vi "Tx Buffered Packet Page.vi"(8 "error in (no error)":errorcluster, 11 "Node Ptr":T6 format="%.0x") -> (0 "error out":errorcluster)   [LabVIEW 2019, in "UDP-Custom-Device System Explorer.lvlib"]
uses:
  UDP-Custom-Device System Explorer.lvlib
  Shared/Types/Shared - Transmit Sim Options.ctl
  Shared/Types/Shared - Transmit Flag Options.ctl
  Shared/Types/Shared - Transmit Echo Options.ctl
  Shared/Types/Shared - Transmit Buffer Options.ctl
  Shared/Types/Shared - Pointer Encoding.ctl
  <vilib>/NI VeriStand/Custom Device API/Custom Device Item Ref.ctl
  Types/Page References/Refs - Tx Buffered Data Packet Page.ctl
  <vilib>/NI VeriStand/Custom Device API/Custom Device API.lvlib
  Property Accessors/Shared Packet Accessors.lvlib
  Property Accessors/Tx Packet Accessors.lvlib
  Property Accessors/Buffered Data Packet.lvlib
  Shared/UDP-Custom-Device Shared.lvlib
panel:
  in  "Config Threading":bool
  in  "Toggle Sim":bool
  in  "Sim Options":T1
  in  "Buffer Options":T2
  in  "Debug Mode":bool caption="Auto-Assign Local NIC"
  in  "Transmit Echo Options":T3
  in  "Transmit Options":T4=enum."One-Shot"
  in  "Port as Channel?":bool caption="Auto-Assign Local NIC"
  in  "Pointer Encoding":T5
  in  "TTL":u16=1
  in  "Multicast?":bool caption="Auto-Assign Local NIC"
  in  "External Buffer?":bool
  in  "Buffer Size (bytes)":u32
  in  "General Header 3":cluster{"Section Name":string}={"Section Name"="Buffer Configuration"}
  in  "Prepend\nHeader?":bool caption="Auto-Assign Local NIC"
  in  "Auto-Assign Local NIC":bool
  in  "Port":u16
  in  "IP Address of Local NIC":string
  in  "General Header 2":cluster{"Section Name":string}={"Section Name"="Network Settings"}
  in  "Destination Port":u16
  in  "IP Address of Destination":string
  in  "Configure Header":bool
  in  "Endianness":u16(ring) items=["big-endian"=0, "little-endian"=2]
  out "Packet ID":i32
  in  "Description":string
  in  "Name":string
  in  "SHDocVw.IWebBrowser":refnum<k7>(container)
  in  "General Header":cluster{"Section Name":string}={"Section Name"="Buffered Transmit Packet"}
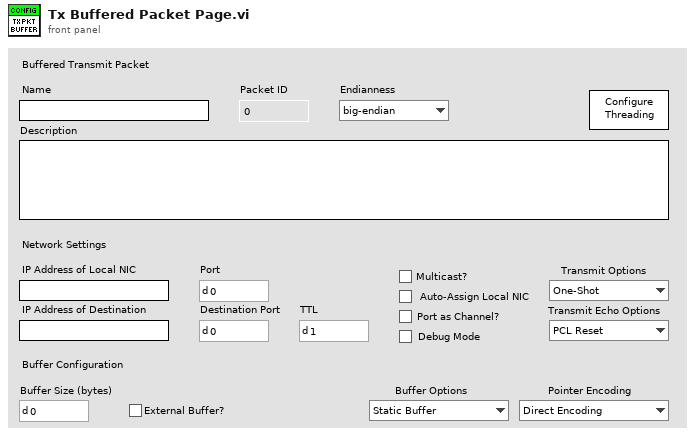
[diagram p1: front panel]
types:
  T1 = typedef "UDP-Custom-Device Shared.lvlib/Shared - Transmit Sim Options.ctl" = enum16{"No Simulation", "Counter", "Full Buffer", "FIFO Test", "FIFO + Port Test"}
  T2 = typedef "UDP-Custom-Device Shared.lvlib/Shared - Transmit Buffer Options.ctl" = enum16{"Static Buffer", "FIFO Buffer", "FIFO Buffer + Port"}
  T3 = typedef "UDP-Custom-Device Shared.lvlib/Shared - Transmit Echo Options.ctl" = enum16{"PCL Reset", "Counter", "Mirror"}
  T4 = typedef "UDP-Custom-Device Shared.lvlib/Shared - Transmit Flag Options.ctl" = enum16{"Always", "One-Shot", "Toggle"}
  T5 = typedef "UDP-Custom-Device Shared.lvlib/Shared - Pointer Encoding.ctl" = enum16{"Direct Encoding", "Conversion Encoding"}
  T6 = typedef "Custom Device API.lvlib/Custom Device Item Ref.ctl" = u64
  T7 = typedef "UDP-Custom-Device System Explorer.lvlib/Refs - Tx Buffered Data Packet Page.ctl" = cluster{"Name":refnum<vi>, "Description":refnum<vi>, "Packet ID":refnum<vi>, "Endianness":refnum<vi>, "Prepend\nHeader?":refnum<vi>, "Configure Header":refnum<vi>, "IP Address of Local NIC":refnum<vi>, "Port":refnum<vi>, "IP Address of Destination":refnum<vi>, "Destination Port":refnum<vi>, "Auto-Assign Local NIC":refnum<vi>, "External Buffer?":refnum<vi>, "Buffer Size (bytes)":refnum<vi>, "Multicast?":refnum<vi>, "TTL":refnum<vi>, "Pointer Encoding":refnum<vi>, "Port as Channel?":refnum<vi>, "Transmit Options":refnum<vi>, "Transmit Echo Options":refnum<vi>, "Debug Mode":refnum<vi>, "Buffer Options":refnum<vi>, "Sim Options":refnum<vi>}
  T8 = enum8{"Enabled", "Disabled", "Disabled and Grayed Out"}
  T9 = typedef "Custom Device API.lvlib/Custom Device Commands.ctl" = enum16{"Default", "Item renamed", "Shutdown", "Dynamic button pressed"}
  T10 = typedef "UDP-Custom-Device System Explorer.lvlib/Thread Configuration.ctl" = cluster{"targetProcessor":i8, "targetPriority":i16, "Synchronization":T11, "loopPeriod":u32, "pclDecimation":u16, "threadManagement":T12}
  T11 = typedef "UDP-Custom-Device System Explorer.lvlib/Thread Sync Reference.ctl" = enum16{"PCL", "Async"}
  T12 = typedef "UDP-Custom-Device Shared.lvlib/Shared - Thread Management.ctl" = enum16{"Untimed (Default)", "Timed (High Priority)"}
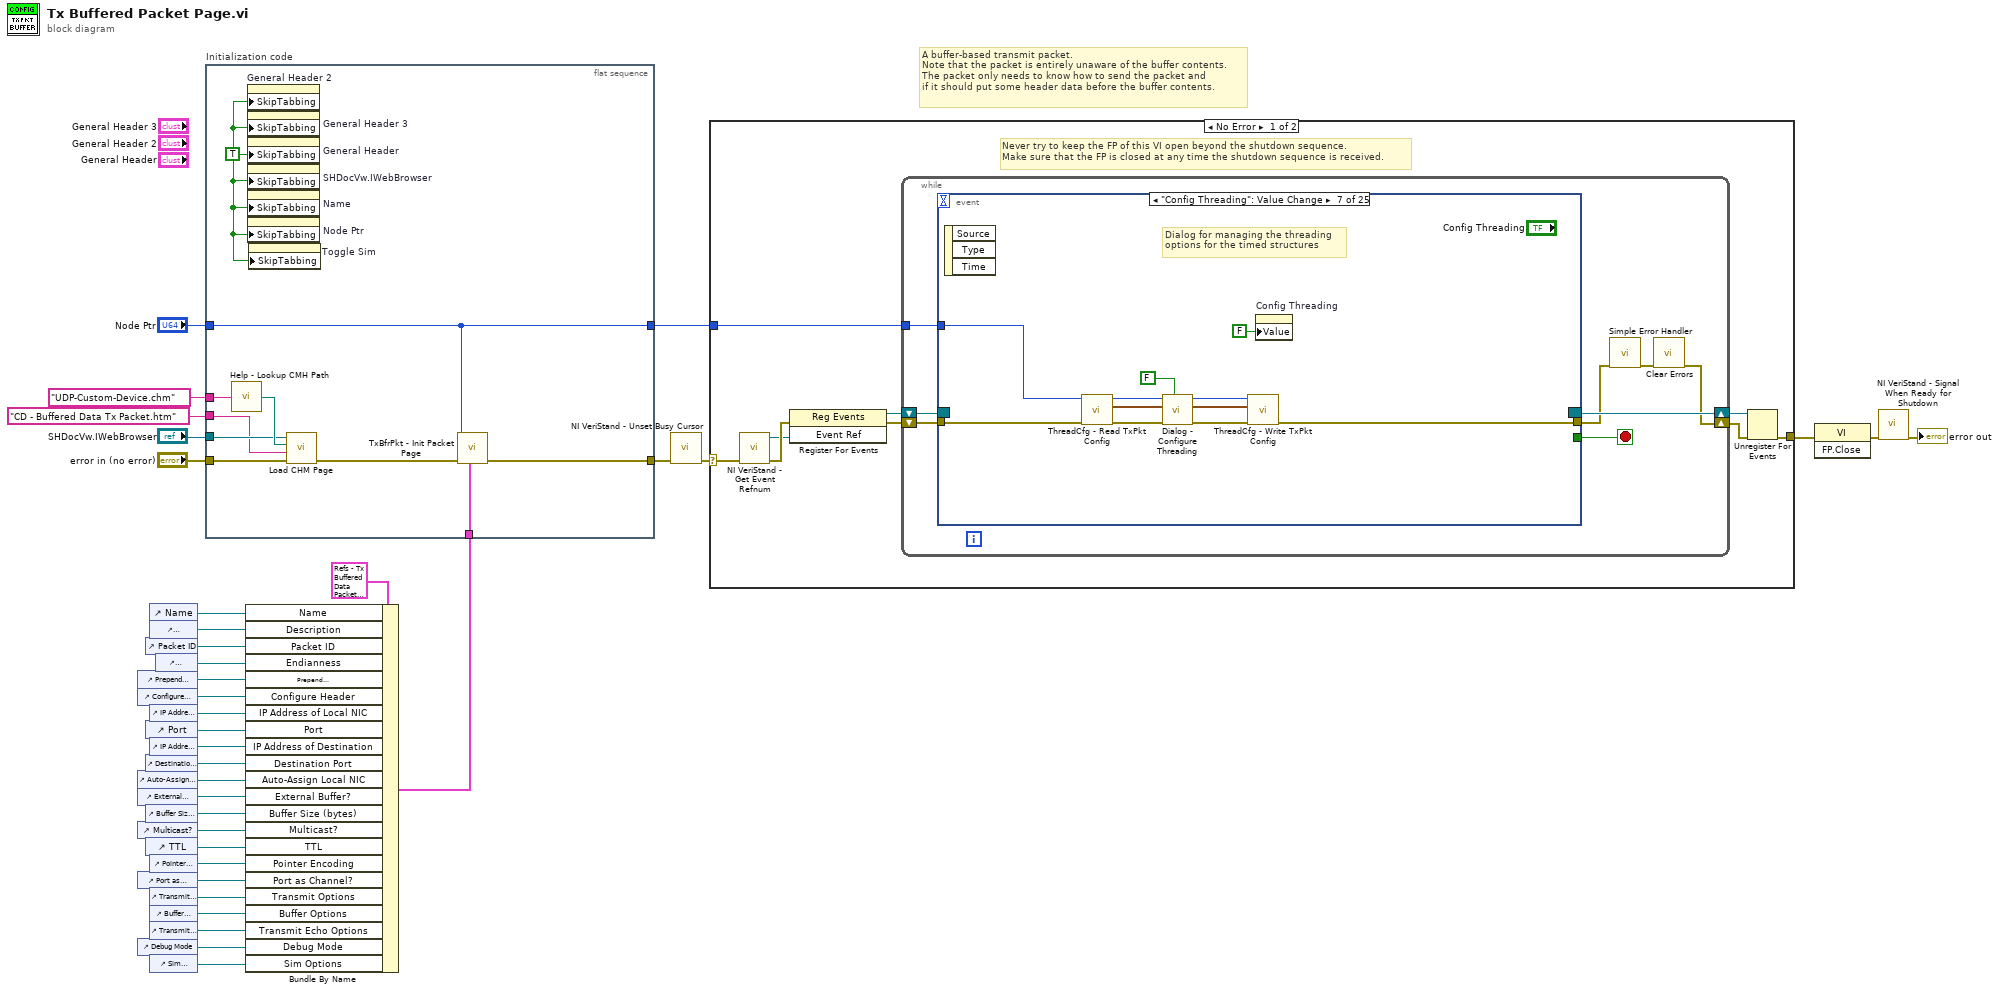
[diagram p0: block diagram]
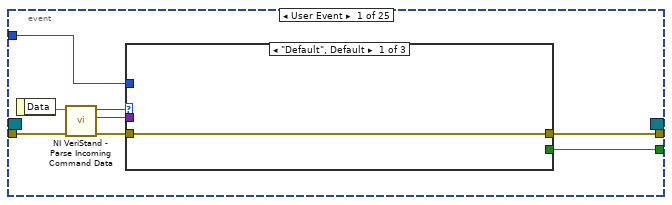
[diagram p2: hidden frame]
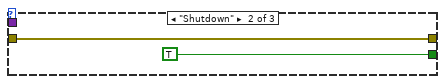
[diagram p3: hidden frame]
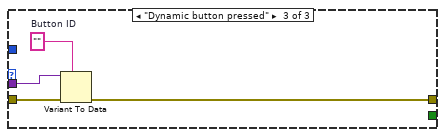
[diagram p4: hidden frame]
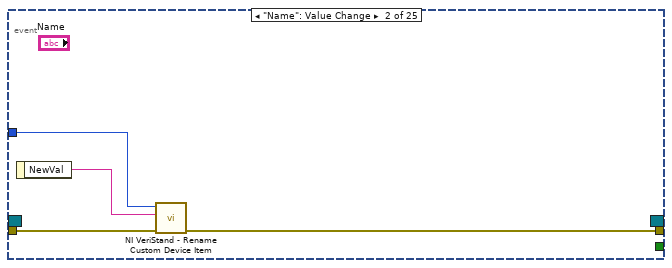
[diagram p5: hidden frame]
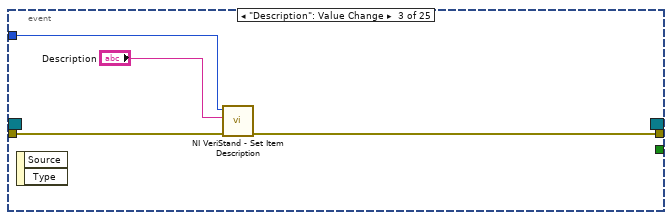
[diagram p6: hidden frame]
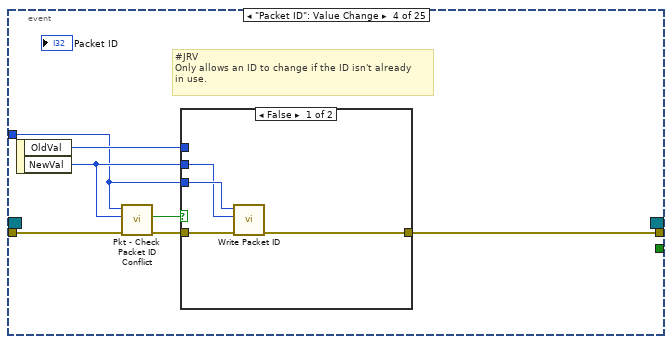
[diagram p7: hidden frame]
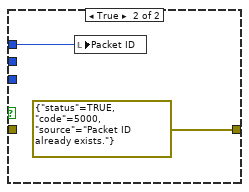
[diagram p8: hidden frame]
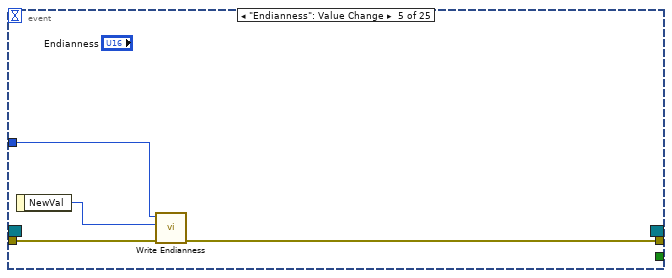
[diagram p9: hidden frame]
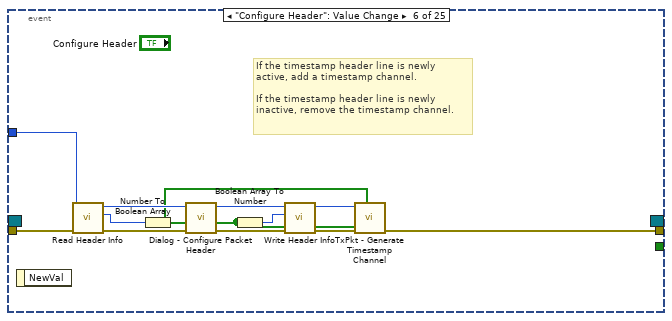
[diagram p10: hidden frame]
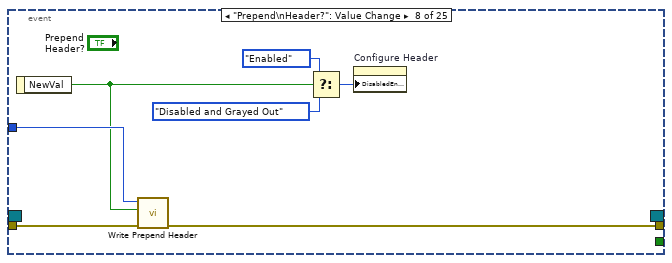
[diagram p11: hidden frame]
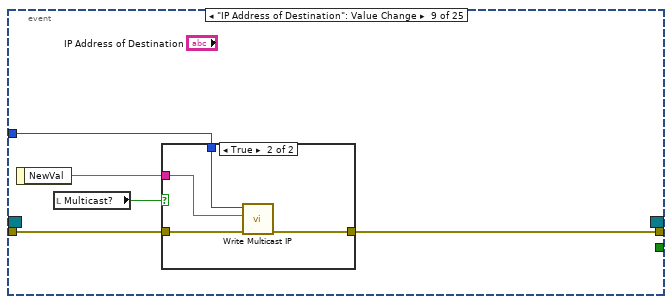
[diagram p12: hidden frame]
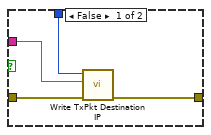
[diagram p13: hidden frame]
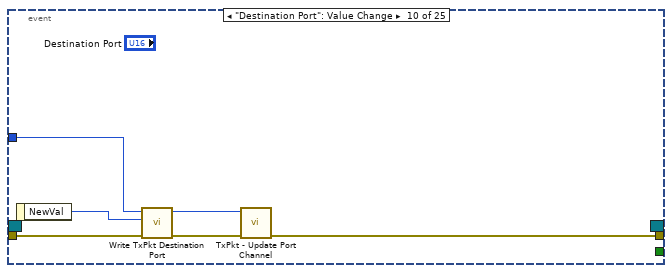
[diagram p14: hidden frame]
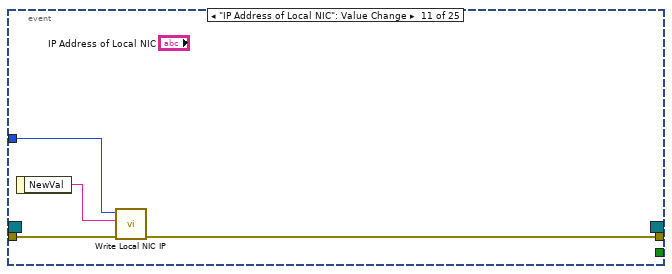
[diagram p15: hidden frame]
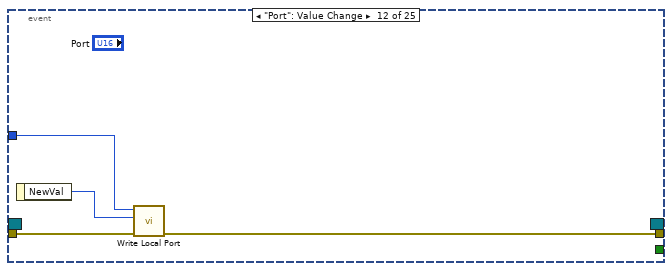
[diagram p16: hidden frame]
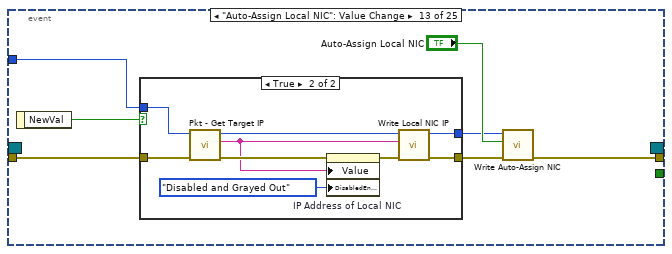
[diagram p17: hidden frame]
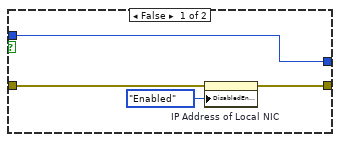
[diagram p18: hidden frame]
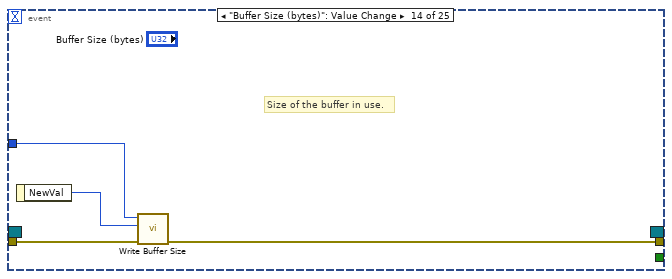
[diagram p19: hidden frame]
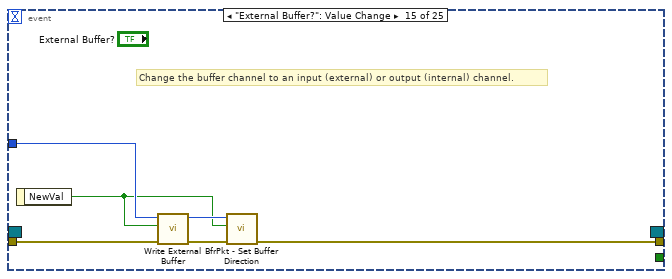
[diagram p20: hidden frame]
diagram:
  # "A buffer-based transmit packet.\nNote that the packet is entirely unaware of the buffer contents.\nThe packet only needs to know how to send the packet and\nif it should put some header data before the buffer contents."
  n1 = control-ref of="Prepend\nHeader?"() -> (w19:refnum<vi>)
  n2 = control-ref of="Configure Header"() -> (w18:refnum<vi>)
  n3 = control-ref of="Auto-Assign Local NIC"() -> (w13:refnum<vi>)
  n4 = control-ref of="External Buffer?"() -> (w12:refnum<vi>)
  n5 = control-ref of="Multicast?"() -> (w9:refnum<vi>)
  n6 = control-ref of="Port as Channel?"() -> (w6:refnum<vi>)
  n7 = control-ref of="Debug Mode"() -> (w3:refnum<vi>)
  n8 = control-ref of="Packet ID"() -> (w21:refnum<vi>)
  n9 = control-ref of="Port"() -> (w16:refnum<vi>)
  n10 = control-ref of="Destination Port"() -> (w14:refnum<vi>)
  n11 = control-ref of="Buffer Size (bytes)"() -> (w11:refnum<vi>)
  n12 = control-ref of="TTL"() -> (w8:refnum<vi>)
  n13 = control-ref of="Name"() -> (w23:refnum<vi>)
  n14 = control-ref of="Description"() -> (w22:refnum<vi>)
  n15 = control-ref of="IP Address of Local NIC"() -> (w17:refnum<vi>)
  n16 = control-ref of="IP Address of Destination"() -> (w15:refnum<vi>)
  n17 = control-ref of="Pointer Encoding"() -> (w7:refnum<vi>)
  n18 = control-ref of="Transmit Options"() -> (w5:refnum<vi>)
  n19 = control-ref of="Buffer Options"() -> (w2:refnum<vi>)
  n20 = control-ref of="Transmit Echo Options"() -> (w4:refnum<vi>)
  n21 = control-ref of="Sim Options"() -> (w1:refnum<vi>)
  n22 = control-ref of="Endianness"() -> (w20:refnum<vi>)
  n23 = flat-sequence "Initialization code" {
    tunnel: "error in (no error)" -> [w44]
    tunnel: "Node Ptr" -> [w40]
    tunnel: [w38] -> w31
    tunnel: [w40] -> w28
    tunnel: "SHDocVw.IWebBrowser" -> [w43]
    tunnel: "CD - Buffered Data Tx Packet.htm" ("CD_CHM_Section") -> [w41]
    tunnel: "UDP-Custom-Device.chm" ("CD_CHM_FileName") -> [w42]
    tunnel: w10 -> [w37]
    frame #0 {
      w36 = TRUE ("Skip When Tabbing")
      n24 = call "Help - Lookup CMH Path.vi"("Main CMH File"=w42) -> ("Compiled CMH Path"=w45:path)
      n25 = property on="General Header 2" class="Clust (strict)"("SkipTabbing"=w36) -> ()  [unwired: 2 in, 2 out]
      n26 = property on="General Header 3" class="Clust (strict)"("SkipTabbing"=w36) -> ()  [unwired: 2 in, 2 out]
      n27 = property on="General Header" class="Clust (strict)"("SkipTabbing"=w36) -> ()  [unwired: 2 in, 2 out]
      n28 = property on="SHDocVw.IWebBrowser" class="AXCont"("SkipTabbing"=w36) -> ()  [unwired: 2 in, 2 out]
      n29 = property on="Name" class="Str"("SkipTabbing"=w36) -> ()  [unwired: 2 in, 2 out]
      n30 = property on="Node Ptr" class="DigNum (strict)"("SkipTabbing"=w36) -> ()  [unwired: 2 in, 2 out]
      n31 = property on="Toggle Sim" class="Bool"("SkipTabbing"=w36) -> ()  [unwired: 2 in, 2 out]
      n32 = call <vilib>:"Load CHM Page.vi"("error in (no error)"=w44, "HTML File"=w41, "Compiled CHM Path"=w45, "Web Browser Reference"=w43) -> ("error out"=w39:errorcluster)  [unwired: 7 in]
      n33 = call "TxBfrPkt - Init Packet Page.vi"("Tx Buffered Data Packet Refs"=w37, "error in (no error)"=w39, "Node Ptr In"=w40) -> ("error out"=w38:errorcluster)  [unwired: 7 in, 1 out]
    }
  }
  n34 = Bundle By Name(cluster=T7 {"Name"=refnum, "Description"=refnum, "Packet ID"=refnum, "Endianness"=refnum, "Prepend\nHeader?"=refnum, "Configure Header"=refnum, "IP Address of Local NIC"=refnum, "Port"=refnum, "IP Address of Destination"=refnum, "Destination Port"=refnum, "Auto-Assign Local NIC"=refnum, "External Buffer?"=refnum, "Buffer Size (bytes)"=refnum, "Multicast?"=refnum, "TTL"=refnum, "Pointer Encoding"=refnum, "Port as Channel?"=refnum, "Transmit Options"=refnum, "Transmit Echo Options"=refnum, "Debug Mode"=refnum, "Buffer Options"=refnum, "Sim Options"=refnum} ("Tx Buffered Data Packet Refs"), "Name"=w23, "Description"=w22, "Packet ID"=w21, "Endianness"=w20, "Prepend\nHeader?"=w19, "Configure Header"=w18, "IP Address of Local NIC"=w17, "Port"=w16, "IP Address of Destination"=w15, "Destination Port"=w14, "Auto-Assign Local NIC"=w13, "External Buffer?"=w12, "Buffer Size (bytes)"=w11, "Multicast?"=w9, "TTL"=w8, "Pointer Encoding"=w7, "Port as Channel?"=w6, "Transmit Options"=w5, "Buffer Options"=w2, "Transmit Echo Options"=w4, "Debug Mode"=w3, "Sim Options"=w1) -> (w10:T7)
  n35 = call <vilib>:"NI VeriStand - Unset Busy Cursor.vi"("error in (no error)"=w31) -> ("error out"=w30:errorcluster)  [unwired: 10 out]
  n36 = case shown="No Error" w30 {
    selector: w30 -> [w46 w254]
    tunnel: [w51 w252] -> w35
    tunnel: w28 -> [w47 _]
    frame No Error {
      # "Never try to keep the FP of this VI open beyond the shutdown sequence.\nMake sure that the FP is closed at any time the shutdown sequence is received."
      n37 = call <vilib>:"NI VeriStand - Get Event Refnum.vi"("error in (no error)"=w46) -> ("error out"=w54:errorcluster, "Event Ref"=w50:refnum<user-event>)  [unwired: 9 out]
      n38 = register-events(error in=w54, w50) -> (reference out=w48:refnum<event-registration>, error out=w49:errorcluster)  [unwired: 1 in]
      n39 = while {
        tunnel: w47 -> [w58]
        shift-right: [w55] -> w52
        shift-left: w49 -> [w61]
        shift-right: [w62] -> w53
        shift-left: w48 -> [w60]
        stop <- w59 stop-if-true
        n40 = event shown="[6] \"Config Threading\": Value Change" {
          selector: w60 -> [_ _ _ _ _ _ _ _ _ _ _ _ _ _ _ _ _ _ _ _ _ _ _ _ _]
          dyn-events: [_ _ _ _ _ _ _ _ _ _ _ _ _ _ _ _ _ _ _ _ _ _ _ _ _] -> w62
          timeout: _ -> [_ _ _ _ _ _ _ _ _ _ _ _ _ _ _ _ _ _ _ _ _ _ _ _ _]
          tunnel: w61 -> [w70 w81 w85 w90 w102 w105 w126 w130 w136 w152 w154 w160 w167 w182 w189 w192 w200 w214 w221 w224 w228 w233 w242 w246 w249]
          tunnel: [w66 _ _ _ _ _ _ _ _ _ _ _ _ _ _ _ _ _ _ _ _ _ _ _ _] -> w59
          tunnel: [w65 w79 w82 w86 w99 w103 w117 w127 w135 w147 w153 w157 w162 w181 w186 w191 w195 w212 w216 w222 w226 w232 w241 w245 w249] -> w57
          tunnel: w58 -> [w64 w80 w84 w87 w101 w104 w125 w129 w138 w150 w155 w158 w165 w184 w190 w193 w201 w215 w219 w225 w229 w234 w244 w248 _]
          event User Event {
            n41 = event-data() -> ("Data"=w69:string)  [unwired: 1 out]
            n42 = call <vilib>:"NI VeriStand - Parse Incoming Command Data.vi"("error in (no error)"=w70, "Incoming data"=w69) -> ("error out"=w68:errorcluster, "Outgoing data"=w63:variant, "Action"=w67:T9)  [unwired: 7 out]
            n43 = case shown="\"Default\", Default" w67 {
              tunnel: w68 -> [w71 w72 w77]
              tunnel: [_ TRUE _] -> w66
              tunnel: [w71 w72 w74] -> w65
              tunnel: w64 -> [_ _ _]
              tunnel: w63 -> [_ _ w76]
              frame "Default", Default {
              }
              frame "Shutdown" {
              }
              frame "Dynamic button pressed" {
                w75 = ""  # Button ID
                n44 = Variant To Data(error in=w77, type=w75, Variant=w76) -> (error out=w74:errorcluster)  [unwired: 1 out]
              }
            }
          }
          event "Name": Value Change {
            n45 = event-data() -> ("NewVal"=w78:string)  [unwired: 1 out]
            n46 = call <vilib>:"NI VeriStand - Rename Custom Device Item.vi"("error in (no error)"=w81, "New Name"=w78, "Item Ref in"=w80) -> ("error out"=w79:errorcluster)  [unwired: 6 in, 2 out]
          }
          event "Description": Value Change {
            n47 = event-data() -> ()  [unwired: 3 out]
            n48 = call <vilib>:"NI VeriStand - Set Item Description.vi"("error in (no error)"=w85, "Description"="Description", "Item Ref in"=w84) -> ("error out"=w82:errorcluster)  [unwired: 6 in, 2 out]
          }
          event "Packet ID": Value Change {
            # "#JRV\nOnly allows an ID to change if the ID isn't already\nin use."
            n49 = event-data() -> ("OldVal"=w89:i32, "NewVal"=w88:i32)  [unwired: 1 out]
            n50 = call "Pkt - Check Packet ID Conflict.vi"("error in (no error)"=w90, "New ID"=w88, "Packet Ref In"=w87) -> ("error out"=w92:errorcluster, "Conflicting ID?"=w91:bool)  [unwired: 7 in]
            n51 = case shown="False" w91 {
              tunnel: w92 -> [w94 _]
              tunnel: w87 -> [w96 _]
              tunnel: [w93 errorcluster {"status"=TRUE, "code"=5000, "source"="Packet ID already exists."} ("error out")] -> w86
              tunnel: w89 -> [_ w97]
              tunnel: w88 -> [w95 _]
              frame False {
                n52 = call "Write Packet ID.vi"("error in (no error)"=w94, "Packet ID"=w95, "Node Ptr"=w96) -> ("error out"=w93:errorcluster)  [unwired: 7 in, 1 out]
              }
              frame True {
                n53 = local write "Packet ID"(w97) -> ()
              }
            }
          }
          event "Endianness": Value Change {
            n54 = event-data() -> ("NewVal"=w100:u16)  [unwired: 1 out]
            n55 = call "Write Endianness.vi"("error in (no error)"=w102, "Endianness"=w100, "Node Ptr"=w101) -> ("error out"=w99:errorcluster)  [unwired: 7 in, 1 out]
          }
          event "Configure Header": Value Change {
            # "If the timestamp header line is newly\nactive, add a timestamp channel.\n\nIf the timestamp header line is newly\ninactive, remove the timestamp channel."
            n56 = event-data() -> ()  [unwired: 2 out]
            n57 = call "Read Header Info.vi"("error in (no error)"=w105, "Node Ptr"=w104) -> ("error out"=w113:errorcluster, "Header Info"=w114:u32, "Node Ptr out"=w115:T6)  [unwired: 7 in]
            n58 = Number To Boolean Array(number=w114) -> (Boolean array=w106:bool[])
            n59 = call "Dialog - Configure Packet Header.vi"("error in (no error)"=w113, "Header Elements In"=w106, "Packet Ref in"=w115) -> ("error out"=w109:errorcluster, "Header Elements Out"=w107:bool[], "Packet Ref out"=w108:T6)  [unwired: 6 in]
            n60 = Boolean Array To Number(Boolean array=w107) -> (number=w110:u32)
            n61 = call "Write Header Info.vi"("error in (no error)"=w109, "Header Info"=w110, "Node Ptr"=w108) -> ("error out"=w112:errorcluster, "Node Ptr out"=w111:T6)  [unwired: 7 in]
            n62 = call "TxPkt - Generate Timestamp Channel.vi"("New Header Config"=w107, "Previous Header Config"=w106, "error in (no error)"=w112, "Packet Ref in"=w111) -> ("error out"=w103:errorcluster)  [unwired: 6 in, 1 out]
          }
          event "Config Threading": Value Change {
            # "Dialog for managing the threading\noptions for the timed structures"
            n63 = event-data() -> ()  [unwired: 4 out]
            n64 = call "ThreadCfg - Read TxPkt Config.vi"("error in (no error)"=w126, "Node Ptr In"=w125) -> ("error out"=w123:errorcluster, "threadOptions"=w121:T10, "Node Ptr Out"=w124:T6)  [unwired: 7 in]
            n65 = call "Dialog - Configure Threading.vi"("rxPacket?"=FALSE, "error in (no error)"=w123, "threadOptions in"=w121, "Packet Ref in"=w124) -> ("error out"=w119:errorcluster, "threadOptions out"=w118:T10, "Packet Ref out"=w120:T6)  [unwired: 4 in]
            n66 = call "ThreadCfg - Write TxPkt Config.vi"("error in (no error)"=w119, "threadOptions"=w118, "Node Ptr In"=w120) -> ("error out"=w117:errorcluster)  [unwired: 7 in, 1 out]
            n67 = property on="Config Threading" class="Bool (strict)"("Value"=FALSE ("Config Threading")) -> ()  [unwired: 2 in, 2 out]
          }
          event "Prepend\nHeader?": Value Change {
            n68 = event-data() -> ("NewVal"=w128:bool)  [unwired: 1 out]
            n69 = call "Write Prepend Header.vi"("error in (no error)"=w130, "Prepend Header"=w128, "Node Ptr"=w129) -> ("error out"=w127:errorcluster)  [unwired: 7 in, 1 out]
            n70 = Select(t=T8."Enabled" ("Disabled"), s=w128, f=T8."Disabled and Grayed Out" ("Disabled")) -> (s? t:f=w131:T8)
            n71 = property on="Configure Header" class="Bool"("DisabledEnum"=w131) -> ()  [unwired: 2 in, 2 out]
          }
          event "IP Address of Destination": Value Change {
            n72 = event-data() -> ("NewVal"=w137:string)  [unwired: 1 out]
            n73 = local read "Multicast?"() -> (w134:bool)
            n74 = case shown="True" w134 {
              tunnel: w138 -> [w142 w146]
              tunnel: w137 -> [w141 w143]
              tunnel: w136 -> [w140 w145]
              tunnel: [w139 w144] -> w135
              frame False {
                n75 = call "Write TxPkt Destination IP.vi"("error in (no error)"=w140, "Destination IP"=w141, "Node Ptr"=w142) -> ("error out"=w139:errorcluster)  [unwired: 7 in, 1 out]
              }
              frame True {
                n76 = call "Write Multicast IP.vi"("error in (no error)"=w145, "Multicast IP Address"=w143, "Node Ptr"=w146) -> ("error out"=w144:errorcluster)  [unwired: 7 in, 1 out]
              }
            }
          }
          event "Destination Port": Value Change {
            n77 = event-data() -> ("NewVal"=w151:u16)  [unwired: 1 out]
            n78 = call "Write TxPkt Destination Port.vi"("error in (no error)"=w152, "Destination Port"=w151, "Node Ptr"=w150) -> ("error out"=w148:errorcluster, "Node Ptr out"=w149:T6)  [unwired: 7 in]
            n79 = call "TxPkt - Update Port Channel.vi"("error in (no error)"=w148, "Packet Ref in"=w149) -> ("error out"=w147:errorcluster)  [unwired: 8 in, 1 out]
          }
          event "IP Address of Local NIC": Value Change {
            n80 = event-data() -> ("NewVal"=w156:string)  [unwired: 1 out]
            n81 = call "Write Local NIC IP.vi"("error in (no error)"=w154, "IP Address of Local NIC"=w156, "Node Ptr"=w155) -> ("error out"=w153:errorcluster)  [unwired: 7 in, 1 out]
          }
          event "Port": Value Change {
            n82 = event-data() -> ("NewVal"=w159:u16)  [unwired: 1 out]
            n83 = call "Write Local Port.vi"("error in (no error)"=w160, "Port"=w159, "Node Ptr"=w158) -> ("error out"=w157:errorcluster)  [unwired: 7 in, 1 out]
          }
          event "Auto-Assign Local NIC": Value Change {
            n84 = event-data() -> ("NewVal"=w166:bool)  [unwired: 1 out]
            n85 = case shown="True" w166 {
              tunnel: w167 -> [w171 w178]
              tunnel: [w169 w173] -> w161
              tunnel: [w168 w172] -> w163
              tunnel: w165 -> [w168 w177]
              frame False {
                n86 = property on="IP Address of Local NIC" class="Str"(error in=w171, "DisabledEnum"=T8."Enabled" ("Disabled")) -> (error out=w169:errorcluster)  [unwired: 1 in, 1 out]
              }
              frame True {
                n87 = call "Pkt - Get Target IP.vi"("error in"=w178, "Item Ref in"=w177) -> ("error out"=w180:errorcluster, "IPAddress"=w175:string, "Item Ref out"=w176:T6)  [unwired: 7 in]
                n88 = property on="IP Address of Local NIC" class="Str"(error in=w180, "Value"=w175, "DisabledEnum"=T8."Disabled and Grayed Out" ("Disabled")) -> (error out=w174:errorcluster)  [unwired: 1 in, 1 out]
                n89 = call "Write Local NIC IP.vi"("error in (no error)"=w174, "IP Address of Local NIC"=w175, "Node Ptr"=w176) -> ("error out"=w173:errorcluster, "Node Ptr out"=w172:T6)  [unwired: 7 in]
              }
            }
            n90 = call "Write Auto-Assign NIC.vi"("error in (no error)"=w161, "Auto-Assign NIC"="Auto-Assign Local NIC", "Node Ptr"=w163) -> ("error out"=w162:errorcluster)  [unwired: 7 in, 1 out]
          }
          event "Buffer Size (bytes)": Value Change {
            # "Size of the buffer in use."
            n91 = event-data() -> ("NewVal"=w183:u32)  [unwired: 1 out]
            n92 = call "Write Buffer Size.vi"("error in (no error)"=w182, "Buffer Size"=w183, "Node Ptr"=w184) -> ("error out"=w181:errorcluster)  [unwired: 7 in, 1 out]
          }
          event "External Buffer?": Value Change {
            # "Change the buffer channel to an input (external) or output (internal) channel."
            n93 = event-data() -> ("NewVal"=w185:bool)  [unwired: 1 out]
            n94 = call "Write External Buffer.vi"("error in (no error)"=w189, "External Buffer"=w185, "Node Ptr"=w190) -> ("error out"=w187:errorcluster, "Node Ptr out"=w188:T6)  [unwired: 7 in]
            n95 = call "BfrPkt - Set Buffer Direction.vi"("error in (no error)"=w187, "External?"=w185, "Node Ptr"=w188) -> ("error out"=w186:errorcluster)  [unwired: 7 in, 1 out]
          }
          event "TTL": Value Change {
            n96 = event-data() -> ("NewVal"=w194:u16)  [unwired: 1 out]
            n97 = call "Write TTL.vi"("error in (no error)"=w192, "TTL"=w194, "Node Ptr"=w193) -> ("error out"=w191:errorcluster)  [unwired: 7 in, 1 out]
          }
          event "Multicast?": Value Change {
            n98 = event-data() -> ("NewVal"=w199:bool)  [unwired: 1 out]
            n99 = call "Write Multicast.vi"("error in (no error)"=w200, "Multicast"=w199, "Node Ptr"=w201) -> ("error out"=w197:errorcluster, "Node Ptr out"=w198:T6)  [unwired: 7 in]
            n100 = case shown="True" w199 {
              tunnel: [w206 w207] -> w195
              tunnel: [w205 w208] -> w196
              tunnel: [w204 w209] -> _
              tunnel: w198 -> [w203 w211]
              tunnel: w197 -> [w202 w210]
              frame False {
                n101 = call "Read TxPkt Destination IP.vi"("error in (no error)"=w202, "Node Ptr"=w203) -> ("error out"=w206:errorcluster, "Destination IP"=w205:string, "Node Ptr out"=w204:T6)  [unwired: 7 in]
              }
              frame True {
                n102 = call "Read Multicast IP.vi"("error in (no error)"=w210, "Node Ptr"=w211) -> ("error out"=w207:errorcluster, "Multicast IP Address"=w208:string, "Node Ptr out"=w209:T6)  [unwired: 7 in]
              }
            }
            n103 = local write "IP Address of Destination"(w196) -> ()
          }
          event Value Change {
            n104 = event-data() -> ("NewVal"=w213:T5)  [unwired: 1 out]
            n105 = call "Write Pointer Encoding.vi"("error in (no error)"=w214, "Pointer Encoding"=w213, "Node Ptr"=w215) -> ("error out"=w212:errorcluster)  [unwired: 7 in, 1 out]
          }
          event "Port as Channel?": Value Change {
            n106 = event-data() -> ("NewVal"=w220:bool)  [unwired: 1 out]
            n107 = call "Write TxPkt Port as Channel.vi"("error in (no error)"=w221, "Port as Channel"=w220, "Node Ptr"=w219) -> ("error out"=w217:errorcluster, "Node Ptr out"=w218:T6)  [unwired: 7 in]
            n108 = call "TxPkt - Handle Port Channel.vi"("error in (no error)"=w217, "Packet Ref in"=w218) -> ("error out"=w216:errorcluster)  [unwired: 8 in, 1 out]
          }
          event Value Change {
            n109 = event-data() -> ("NewVal"=w223:T4)  [unwired: 1 out]
            n110 = call "Write TxPkt Transmit Option.vi"("error in (no error)"=w224, "Transmit Options"=w223, "Node Ptr"=w225) -> ("error out"=w222:errorcluster)  [unwired: 7 in, 1 out]
          }
          event Value Change {
            n111 = event-data() -> ("NewVal"=w227:T3)  [unwired: 1 out]
            n112 = call "Write TxPkt Transmit Echo Option.vi"("error in (no error)"=w228, "Transmit Echo Options"=w227, "Node Ptr"=w229) -> ("error out"=w226:errorcluster)  [unwired: 7 in, 1 out]
          }
          event Value Change {
            n113 = event-data() -> ("NewVal"=w230:T2)  [unwired: 1 out]
            n114 = call "Write Tx Buffer Option.vi"("error in (no error)"=w233, "Buffer Option"=w230, "Node Ptr"=w234) -> ("error out"=w231:errorcluster)  [unwired: 7 in, 1 out]
            n115 = case shown="\"FIFO Buffer + Port\"" w230 {
              tunnel: [w236 w238 w240] -> w232
              tunnel: w231 -> [w236 w238 w240]
              frame "Static Buffer", Default {
                n116 = property on="Destination Port" class="DigNum (strict)"("DisabledEnum"=T8."Enabled" ("Disabled")) -> ()  [unwired: 2 in, 2 out]
              }
              frame "FIFO Buffer" {
                n117 = property on="Destination Port" class="DigNum (strict)"("DisabledEnum"=T8."Enabled" ("Disabled")) -> ()  [unwired: 2 in, 2 out]
              }
              frame "FIFO Buffer + Port" {
                n118 = property on="Destination Port" class="DigNum (strict)"("DisabledEnum"=T8."Disabled and Grayed Out" ("Disabled")) -> ()  [unwired: 2 in, 2 out]
              }
            }
          }
          event "Debug Mode": Value Change {
            n119 = event-data() -> ("NewVal"=w243:bool)  [unwired: 1 out]
            n120 = call "Write Debug Mode.vi"("error in (no error)"=w242, "Debug Mode"=w243, "Node Ptr"=w244) -> ("error out"=w241:errorcluster)  [unwired: 7 in, 1 out]
          }
          event Value Change {
            n121 = event-data() -> ("NewVal"=w247:T1)  [unwired: 1 out]
            n122 = call "Write Tx Sim Option.vi"("error in (no error)"=w246, "Sim Option"=w247, "Node Ptr"=w248) -> ("error out"=w245:errorcluster)  [unwired: 7 in, 1 out]
          }
          event "Toggle Sim": Value Change {
            n123 = event-data() -> ()  [unwired: 2 out]
            n124 = property on="Sim Options" class="Enum (strict)"() -> ("Visible"=w251:bool)  [unwired: 2 in, 2 out]
            n125 = Not(x=w251) -> (.not. x?=w250:bool)
            n126 = property on="Sim Options" class="Enum (strict)"("Visible"=w250) -> ()  [unwired: 2 in, 2 out]
          }
        }
        n127 = call <vilib>:"Simple Error Handler.vi"("error in (no error)"=w57) -> ("error out"=w56:errorcluster)  [unwired: 1 in, 7 out]
        n128 = call <vilib>:"Clear Errors.vi"("error in (no error)"=w56) -> ("error out"=w55:errorcluster)  [unwired: 1 in, 5 out]
      }
      n129 = Unregister For Events(event registration refnum=w53, error in=w52) -> (error out=w51:errorcluster)
    }
    frame Error {
      n130 = call <vilib>:"Simple Error Handler.vi"("error in (no error)"=w254) -> ("error out"=w253:errorcluster)  [unwired: 1 in, 7 out]
      n131 = call <vilib>:"Clear Errors.vi"("error in (no error)"=w253) -> ("error out"=w252:errorcluster)  [unwired: 1 in, 5 out]
    }
  }
  n132 = invoke class="VI" method="FP.Close"(error in=w35) -> (error out=w34:errorcluster)  [unwired: 2 in, 2 out]
  n133 = call <vilib>:"NI VeriStand - Signal When Ready for Shutdown.vi"("error in (no error)"=w34) -> ("error out"=→"error out":errorcluster)  [unwired: 10 out]
